vi "Erreur executable (SubVI).vi"(8 "error in (no error)":errorcluster) -> (0 "error out":errorcluster)   [LabVIEW 2015]
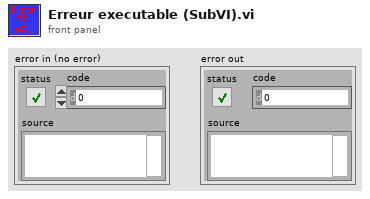
[diagram p1: front panel]
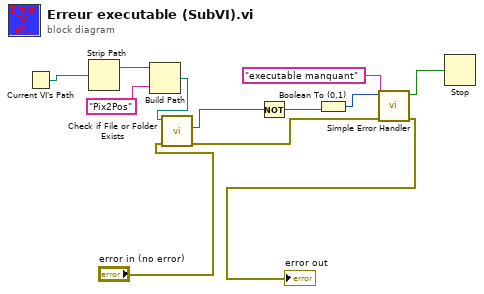
[diagram p0: block diagram]
diagram:
  n1 = Current VI's Path() -> (path=w2:path)
  n2 = Strip Path(path=w2) -> (stripped path=w3:path)  [unwired: 1 out]
  n3 = Build Path(base path=w3, name or relative path="Pix2Pos") -> (appended path=w5:path)
  n4 = call <vilib>:"Check if File or Folder Exists.vi"("error in (no error)"="error in (no error)", "path"=w5) -> ("error out"=w11:errorcluster, "file or folder exists?"=w10:bool)  [unwired: 7 in, 1 out]
  n5 = Not(x=w10) -> (.not. x?=w9:bool)
  n6 = Boolean To (0,1)(Boolean=w9) -> (0, 1=w7:i16)
  n7 = call <vilib>:"Simple Error Handler.vi"("error code (no error:0)"=w7, "error source (\" \")"="executable manquant" ("error source (\" \")"), "error in (no error)"=w11) -> ("error?"=w8:bool, "error out"=→"error out":errorcluster)  [unwired: 2 in, 3 out]
  n8 = Stop(stop? (T)=w8) -> ()
